vi "Log 2D Data.vi"(8 "error in (no error)":errorcluster, 10 "2D Data with Headers":string[][](array[string]), 11 "SLL Spreadsheet Logger in":refnum<class "SLL CSV Logger.lvclass">) -> (0 "error out":errorcluster, 3 "SLL Spreadsheet Logger out":refnum<class "SLL CSV Logger.lvclass">)   [LabVIEW 2016, in "SLL Spreadsheet.lvlib" / "SLL CSV Logger.lvclass"]
doc: "Provide a 2D Data with Headers to log. \n\nThe headers can be in any order and new headers can also be present, which were not provided previously."
uses:
  SLL CSV Logger.lvclass
  SLL CSV Logger.lvclass/SLL CSV Logger.ctl
  SLL Spreadsheet.lvlib
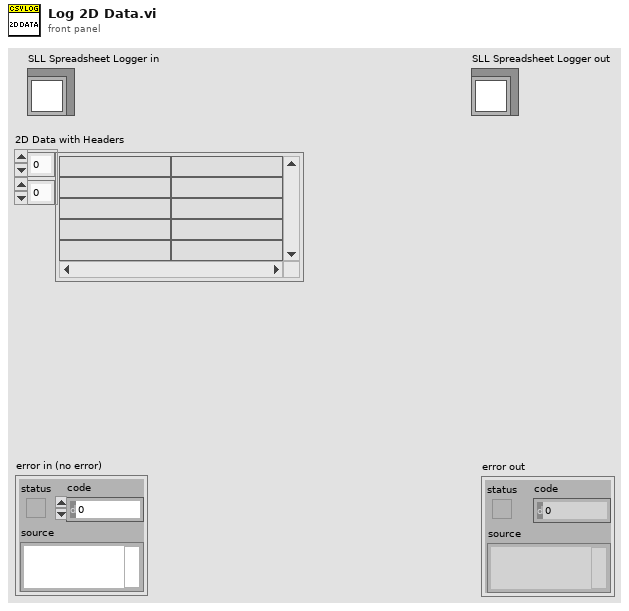
[diagram p1: front panel]
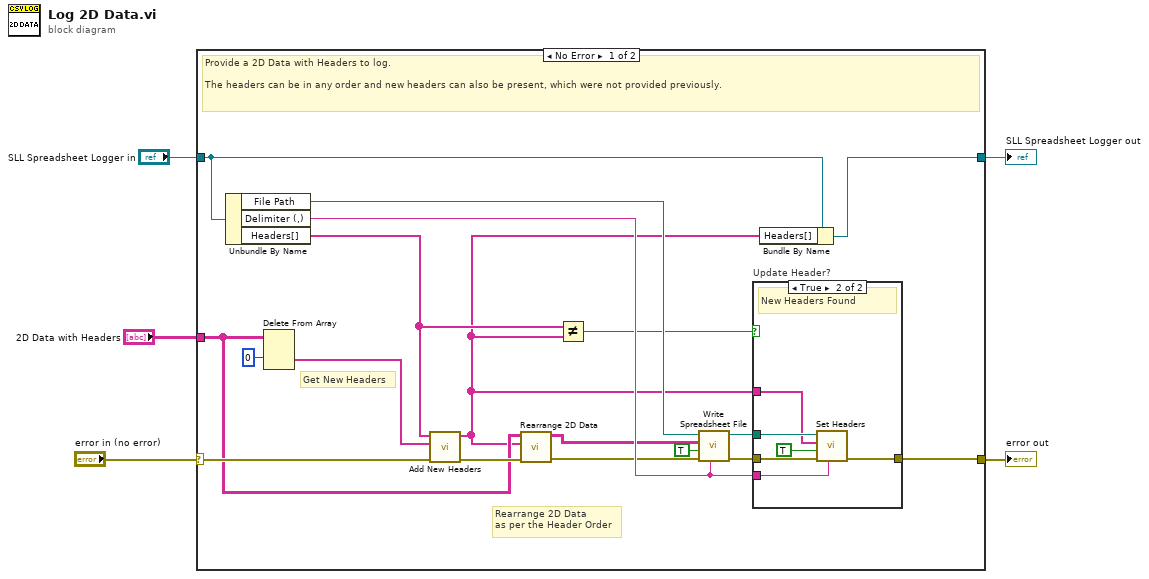
[diagram p0: block diagram]
diagram:
  n1 = case shown="No Error" "error in (no error)" {
    selector: "error in (no error)" -> [w13 w32]
    tunnel: [w15 w32] -> w4
    tunnel: [w22 w31] -> w2
    tunnel: "SLL Spreadsheet Logger in" -> [w23 w31]
    tunnel: "2D Data with Headers" -> [w8 _]
    frame No Error {
      # "Rearrange 2D Data\nas per the Header Order"
      # "Get New Headers"
      # "Provide a 2D Data with Headers to log. \n\nThe headers can be in any order and new headers can also be present, which were not provided previously."
      n2 = Unbundle By Name(w23) -> ("File Path"=w21:path, "Delimiter (,)"=w17:string, "Headers[]"=w14:string[])
      n3 = Delete From Array(array=w8, index (row)=0) -> (deleted portion=w11:string[])  [unwired: 2 in, 1 out]
      n4 = call "Add New Headers.vi"("error in (no error)"=w13, "Incoming Headers[]"=w11, "Existing Headers[]"=w14) -> ("error out"=w10:errorcluster, "Headers[] Out"=w7:string[])  [unwired: 7 in]
      n5 = call "Rearrange 2D Data.vi"("error in (no error)"=w10, "All Headers Order"=w7, "2D Data with Headers In"=w8) -> ("error out"=w9:errorcluster, "2D Data Out without Headers[]"=w6:string[][])  [unwired: 7 in]
      n6 = Not Equal?(x=w14, y=w7) -> (x != y?=w16:bool)
      n7 = call "Write Spreadsheet File.vi"("Delimiter (tab)"=w17, "error in (no error)"=w9, "Append to File? (F)"=TRUE, "2D String[][]"=w6, "File Path"=w21) -> ("error out"=w18:errorcluster, "File Path dup"=w19:path)  [unwired: 5 in]
      n8 = case "Update Header?" shown="True" w16 {
        tunnel: w19 -> [_ w30]
        tunnel: w18 -> [w24 w29]
        tunnel: w7 -> [_ w28]
        tunnel: w17 -> [_ w26]
        tunnel: [w24 w25] -> w15
        frame False {
        }
        frame True {
          # "New Headers Found"
          n9 = call "Set Headers.vi"("Delimiter (,)"=w26, "error in (no error)"=w29, "Update Existing? (T)"=TRUE ("Update Existing? (F)"), "Headers[]"=w28, "File Path"=w30) -> ("error out"=w25:errorcluster)  [unwired: 5 in, 1 out]
        }
      }
      n10 = Bundle By Name(cluster=w23, "Headers[]"=w7) -> (w22:refnum<class "SLL CSV Logger.lvclass">)
    }
    frame Error {
    }
  }
  "error out" <- w4
  "SLL Spreadsheet Logger out" <- w2
